vi "Read Values DVR.vi"(8 "error in (no error)":errorcluster, 11 "DAQmx - Analog Input Single Sample in":refnum<class "DAQmx - Analog Input Single Sample.lvclass">) -> (0 "error out":errorcluster, 2 "Values DVR":refnum<data-value>, 3 "DAQmx - Analog Input Single Sample out":refnum<class "DAQmx - Analog Input Single Sample.lvclass">)   [LabVIEW 2021, in "DAQmx - Analog Input Single Sample.lvclass"]
uses:
  DAQmx - Analog Input Single Sample.lvclass
  DAQmx - Analog Input Single Sample.lvclass/DAQmx - Analog Input Single Sample.ctl
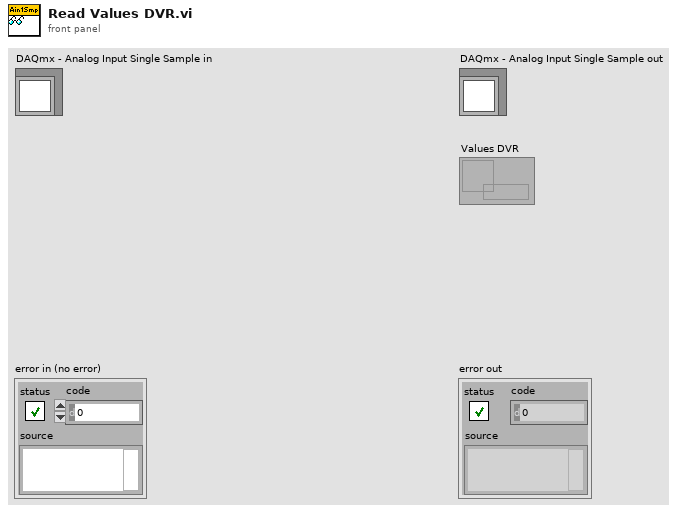
[diagram p1: front panel]
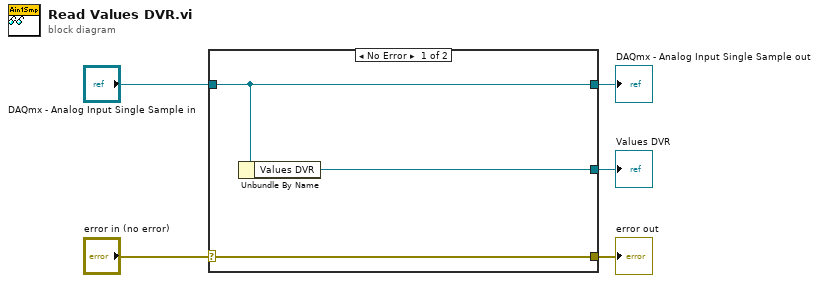
[diagram p0: block diagram]
diagram:
  n1 = case shown="No Error" "error in (no error)" {
    selector: "error in (no error)" -> [w8 w9]
    tunnel: [w8 w9] -> w4
    tunnel: [w7 w10] -> w2
    tunnel: "DAQmx - Analog Input Single Sample in" -> [w7 w10]
    tunnel: [w6 _] -> w1
    frame No Error {
      n2 = Unbundle By Name(w7) -> ("Values DVR"=w6:refnum<data-value>)
    }
    frame Error {
    }
  }
  "error out" <- w4
  "DAQmx - Analog Input Single Sample out" <- w2
  "Values DVR" <- w1
